vi "getDI.vi"(8 "错误输入（无错误）":errorcluster, 10 "channel":i32) -> (0 "错误输出":errorcluster, 3 "result":bool=TRUE)   [LabVIEW 2013]
panel:
  in  "buff":dbl format="%#_13g"
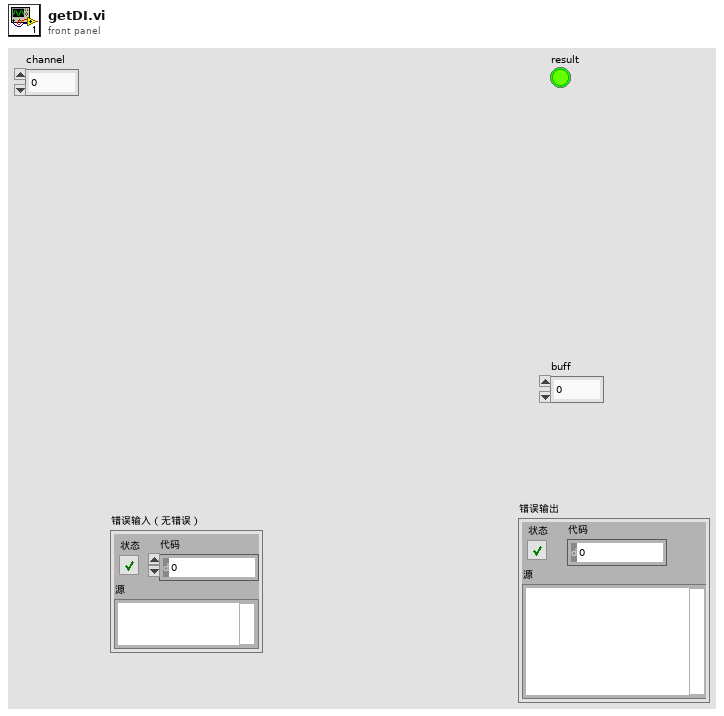
[diagram p1: front panel]
types:
  T1 = cluster{"cmd":string, "channel":i32, "value":dbl, "on/off":bool, "return value":refnum<vi>}
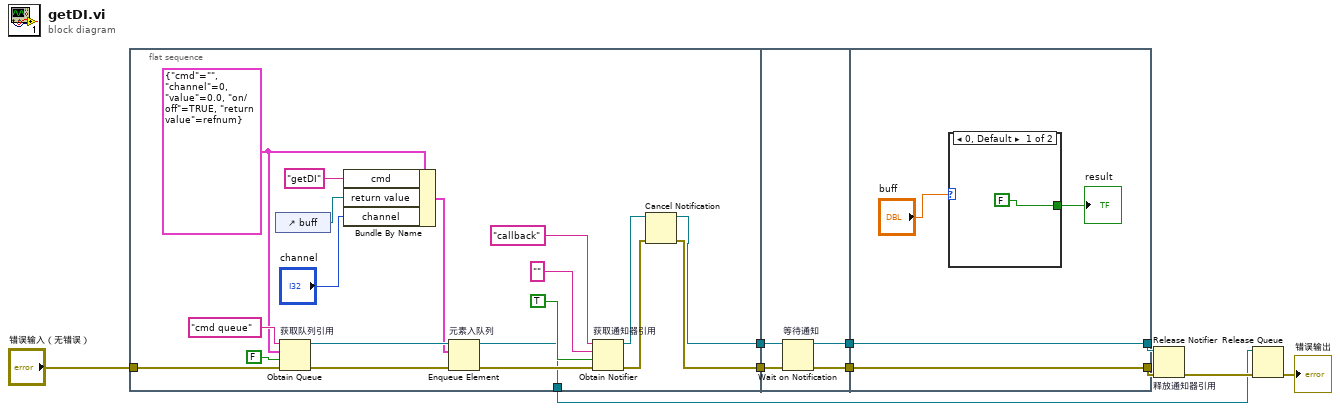
[diagram p0: block diagram]
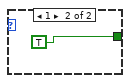
[diagram p2: hidden frame]
diagram:
  n1 = flat-sequence {
    tunnel: [w11] -> w10
    tunnel: [w13] -> w9
    tunnel: "错误输入（无错误）" -> [w24]
    tunnel: [w15] -> w2
    tunnel: w10 -> [w33]
    tunnel: w9 -> [w32]
    tunnel: [w31] -> w8
    tunnel: [w30] -> w6
    tunnel: w8 -> [w37]
    tunnel: [w37] -> w7
    tunnel: w6 -> [w36]
    tunnel: [w36] -> w5
    frame #0 {
      w18 = T1 {"cmd"="", "channel"=0, "value"=0.0, "on/off"=TRUE, "return value"=refnum}
      n2 = control-ref of="buff"() -> (w19:refnum<vi>)
      n3 = Obtain Queue "获取队列引用"(name (unnamed)="cmd queue" ("名称（未命名）"), element data type=w18, create if not found? (T)=FALSE ("如未找到是否创建？(T)"), error in (no error)=w24) -> (queue out=w20:refnum<queue>, error out=w21:errorcluster)  [unwired: 1 in, 1 out]
      n4 = Bundle By Name(cluster=w18, "cmd"="getDI", "return value"=w19, "channel"="channel") -> (w17:T1)
      n5 = Enqueue Element "元素入队列"(queue=w20, element=w17, error in (no error)=w21) -> (queue out=w15:refnum<queue>, error out=w16:errorcluster)  [unwired: 1 in, 1 out]
      n6 = Obtain Notifier "获取通知器引用"(name (unnamed)="callback" ("名称（未命名）"), notification data type="", create if not found? (T)=TRUE ("如未找到是否创建？(T)"), error in (no error)=w16) -> (notifier out=w12:refnum<notifier>, error out=w14:errorcluster)  [unwired: 1 out]
      n7 = Cancel Notification(0:w12, 3:w14) -> (8:w11:refnum<notifier>, 11:w13:errorcluster)  [unwired: 1 out]
    }
    frame #1 {
      n8 = Wait on Notification "等待通知"(notifier=w33, error in (no error)=w32) -> (notifier out=w31:refnum<notifier>, error out=w30:errorcluster)  [unwired: 2 in, 2 out]
    }
    frame #2 {
      n9 = case shown="0, Default" "buff" {
        tunnel: [FALSE TRUE] -> w34
        frame 0, Default {
        }
        frame 1 {
        }
      }
      "result" <- w34
    }
  }
  n10 = Release Notifier "释放通知器引用"(notifier=w7, error in (no error)=w5) -> (error out=w3:errorcluster)  [unwired: 1 in, 2 out]
  n11 = Release Queue(queue=w2, error in (no error)=w3) -> (error out=→"错误输出":errorcluster)  [unwired: 1 in, 2 out]
